vi "DATE_FIILE.vi"() -> ()   [LabVIEW 2020]
panel:
  out "Filename":string
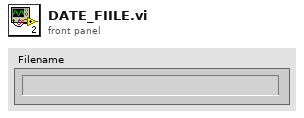
[diagram p1: front panel]
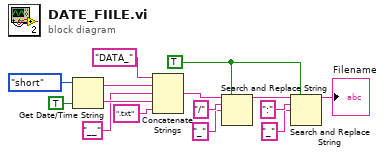
[diagram p0: block diagram]
diagram:
  w7 = TRUE ("replace all? (F)")
  n1 = Get Date/Time String(date format (0)=enum16{"short", "long", "abbreviated"}."short", want seconds? (F)=TRUE) -> (date string=w15:string, time string=w5:string)  [unwired: 1 in]
  n2 = Concatenate Strings("DATA_" ("string"), w15, "__" ("string"), w5, ".txt") -> (w13:string)
  n3 = Search and Replace String(replace all?=w7, input string=w13, search string="/", replace string="_" ("replace string (\"\")")) -> (result string=w10:string)  [unwired: 4 in, 3 out]
  n4 = Search and Replace String(replace all?=w7, input string=w10, search string=":", replace string="_" ("replace string (\"\")")) -> (result string=→"Filename":string)  [unwired: 4 in, 3 out]
